vi "Graph Builder GUI - 4Dsupported.vi"() -> ()   [LabVIEW 2019]
uses:
  AxisMenu--Enum.ctl
  <vilib>/Utility/file.llb/Read Delimited Spreadsheet (string).vi
panel:
  in  "Axis Menus 2":T1={"Axis Menu 1"=1, "Axis Menu 2"=3, "Axis Menu 3"=0, "Axis Menu 4"=7, "Axis Menu 5"=9, "Axis Menu 6"=0, "Axis Menu 7"=0, "Axis Menu 8"=0, "Axis Menu 9"=4, "Axis Menu 10"=2, "Axis Menu 11"=0, "Axis Menu 12"=0} {"Axis Menu 12" items=["test", "what", "ok"]; "Axis Menu 11" items=["<Ignore>", "<X Axis>", "<Y Axis>", "<Color Axis>", "<Time Axis>", "<Supra-X Scroll>", "<Supra-Y Scroll>", "0.130833", "0.130832", "0.130830", "0.130828", "0.130824", "0.130816", "0.130803", "0.130780", "0.130738", "0.130664", "0.130532", "0.148603", "0.148602", "0.148601", "0.148600", "0.148597", "0.148593", "0.148584", "0.148569", "0.148542", "0.148495", "0.148411", "0.148262", "0.169040", "0.169039", "0.169038", "0.169036", "0.169033", "0.169028", "0.169018", "0.169001", "0.168971", "0.168917", "0.168821", "0.168651", "0.191677", "0.191676", "0.191675", "0.191674", "0.191672", "0.191669", "0.191663", "0.191652", "0.191633", "0.191598", "0.191537", "0.191429", "0.191236", "0.216833", "0.216832", "0.216831", "0.216828", "0.216824", "0.216818", "0.216805", "0.216783", "0.216745", "0.216676", "0.216553", "0.216335", "0.247333", "0.247332", "0.247330", "0.247328", "0.247323", "0.247315", "0.247301", "0.247276", "0.247232", "0.247153", "0.247013", "0.246764", "0.282147", "0.282146", "0.282145", "0.282143", "0.282140", "0.282135", "0.282126", "0.282110", "0.282082", "0.282031", "0.281941", "0.281782", "0.281498", "0.132273", "0.132272", "0.132270", "0.132268", "0.132264", "0.132256", "0.132243", "0.132219", "0.132177", "0.132102", "0.131969", "0.150477", "0.150476", "0.150475", "0.150473"]; "Axis Menu 10" items=["<Ignore>", "<X Axis>", "<Y Axis>", "<Color Axis>", "<Time Axis>", "<Supra-X Scroll>", "<Supra-Y Scroll>", " 0.000001", " 0.000100", " 0.000178", " 0.000316", " 0.000562", " 0.001000", " 0.001778", " 0.003162", " 0.005623", " 0.010000", " 0.017783", " 0.031623", " 0.056234", " 0.100000", " 0.177828", " 0.316228", " 0.562341", " 1.000000", " 1.778279", " 3.162278", " 5.623413", " 10.000000"]; "Axis Menu 9" items=["<Ignore>", "<X Axis>", "<Y Axis>", "<Color Axis>", "<Time Axis>", "<Supra-X Scroll>", "<Supra-Y Scroll>", "0.000000", "0.000009", "0.000008", "0.000007", "0.000027", "0.000026", "0.000024", "0.000023", "0.000021", "0.000020", "0.000019", "0.009968", "0.011864", "0.014201", "0.017147", "0.020963", "0.026238", "0.033996", "0.021918", "0.023911", "0.025861", "0.026573", "0.030301", "0.047063", "0.057440", "0.023065", "0.025858", "0.047064", "0.023066", "0.030300", "0.043640", "0.041839", "0.040309", "0.039572", "0.040076", "0.047266", "0.070634", "0.043275", "0.041840", "0.040209", "0.039424", "0.047267", "0.040077", "0.068931", "0.041841", "0.039425", "0.041842", "0.040188", "0.057164", "0.055857", "0.053803", "0.064045", "0.062643", "0.079336", "0.084486", "0.057166", "0.055755", "0.053805", "0.062858", "0.062644", "0.079293", "0.084489", "0.057168", "0.055757", "0.053806", "0.062859", "0.084490", "0.057169", "0.054590", "0.053808", "0.062861", "0.062645", "0.084487", "0.057171", "0.054591", "0.053809", "0.079294", "0.084488", "0.094881", "0.146114", "0.159443", "0.157470", "0.165770", "0.210973", "0.222273", "0.083860", "0.145194", "0.159522", "0.153900", "0.165858", "0.198740", "0.221867", "0.083920", "0.145042", "0.159585", "0.153985", "0.165272", "0.198828", "0.221738", "0.083830"]; "Axis Menu 8" items=["<Ignore>", "<X Axis>", "<Y Axis>", "<Color Axis>", "<Time Axis>", "<Supra-X Scroll>", "<Supra-Y Scroll>", "0.000100", "0.115754", "0.118456", "0.121668", "0.125585", "0.130445", "0.136809", "0.145589", "0.115756", "0.118488", "0.121728", "0.125684", "0.130588", "0.137092", "0.145948", "0.115755", "0.118457", "0.121725", "0.130587", "0.137090", "0.145946", "0.130586", "0.145945", "0.125683", "0.121724", "0.130585", "0.137089", "0.116301", "0.118995", "0.122196", "0.125991", "0.130788", "0.137250", "0.146371", "0.116271", "0.118994", "0.122182", "0.125976", "0.130786", "0.137248", "0.146369", "0.125975", "0.130785", "0.137246", "0.146312", "0.118993", "0.125974", "0.137245", "0.122177", "0.130784", "0.116417", "0.119132", "0.122246", "0.126270", "0.131185", "0.137848", "0.146643", "0.119115", "0.122243", "0.126211", "0.131183", "0.137836", "0.146636", "0.116416", "0.119113", "0.126209", "0.137835", "0.146632", "0.119058", "0.122241", "0.126208", "0.131182", "0.146628", "0.116415", "0.119057", "0.126207", "0.137833", "0.146627", "0.119561", "0.123571", "0.127830", "0.132135", "0.138249", "0.146742", "0.157620", "0.119287", "0.123423", "0.127757", "0.131884", "0.138171", "0.146298", "0.157507", "0.119274", "0.123353", "0.127748", "0.131866", "0.138073", "0.146278", "0.157425", "0.119234"]; "Axis Menu 7" items=["<Ignore>", "<X Axis>", "<Y Axis>", "<Color Axis>", "<Time Axis>", "<Supra-X Scroll>", "<Supra-Y Scroll>", "39250.000000", "44581.000000", "50712.000000", "57503.000000", "65050.000000", "74200.000000", "84644.000000", "39682.000000", "45143.000000", "51191.000000", "57807.000000", "65518.000000", "74460.000000", "84954.000000", "39551.000000", "45105.000000", "51201.000000", "57817.000000", "65260.000000", "74304.000000", "84692.000000", "39877.000000", "45240.000000", "51394.000000", "58153.000000", "65752.000000", "74616.000000", "85111.000000", "39561.000000", "45096.000000", "51328.000000", "57851.000000", "65269.000000", "74275.000000", "84761.000000", "39440.000000", "44789.000000", "50739.000000", "57377.000000", "64848.000000", "73617.000000", "84298.000000", "39725.000000", "45219.000000", "51293.000000", "57890.000000", "65468.000000", "74547.000000", "85034.000000", "39753.000000", "45230.000000", "51299.000000", "58146.000000", "65861.000000", "74815.000000", "85419.000000", "39615.000000", "45004.000000", "51015.000000", "57909.000000", "65576.000000", "74531.000000", "85128.000000", "39612.000000", "44999.000000", "51011.000000", "65574.000000", "74528.000000", "85125.000000", "44998.000000", "65573.000000", "74527.000000", "85124.000000", "44997.000000", "51010.000000", "57907.000000", "65572.000000", "51009.000000", "65571.000000", "74526.000000", "39556.000000", "45059.000000", "51216.000000", "57906.000000", "65525.000000", "74511.000000", "85154.000000", "45056.000000", "51213.000000", "57901.000000", "65522.000000", "74506.000000", "85151.000000", "45055.000000", "57899.000000", "65519.000000", "74502.000000", "85145.000000", "45054.000000", "57897.000000"]; "Axis Menu 6" items=["<Ignore>", "<X Axis>", "<Y Axis>", "<Color Axis>", "<Time Axis>", "<Supra-X Scroll>", "<Supra-Y Scroll>", "1.000", "1.500", "2.000", "2.500", "3.000"]; "Axis Menu 5" items=["<Ignore>", "<X Axis>", "<Y Axis>", "<Color Axis>", "<Time Axis>", "<Supra-X Scroll>", "<Supra-Y Scroll>", "0.900", "0.950", "1.000", "1.050", "1.100", "1.150", "1.200"]; "Axis Menu 4" items=["<Ignore>", "<X Axis>", "<Y Axis>", "<Color Axis>", "<Time Axis>", "<Supra-X Scroll>", "<Supra-Y Scroll>", "300000"]; "Axis Menu 3" items=["<Ignore>", "<X Axis>", "<Y Axis>", "<Color Axis>", "<Time Axis>", "<Supra-X Scroll>", "<Supra-Y Scroll>", "0.000000E+0", "1.250000E-1", "2.500000E-1", "5.000000E-1", "1.600000E+1", "4.000000E+0", "8.000000E+0", "1.000000E+0", "2.000000E+0"]; "Axis Menu 2" items=["<Ignore>", "<X Axis>", "<Y Axis>", "<Color Axis>", "<Time Axis>", "<Supra-X Scroll>", "<Supra-Y Scroll>", "1.000000E-10", "1.000000E-1", "2.000000E-1", "3.000000E-1", "4.000000E-1", "5.000000E-1", "6.000000E-1", "7.000000E-1", "8.000000E-1", "9.000000E-1", "1.000000E+0", "1.100000E+0", "1.200000E+0", "1.300000E+0", "1.400000E+0", "1.500000E+0", "1.600000E+0", "1.700000E+0", "1.800000E+0", "1.900000E+0", "2.000000E+0", "3.000000E+0", "4.000000E+0", "5.000000E+0"]; "Axis Menu 1" items=["<Ignore>", "<X Axis>", "<Y Axis>", "<Color Axis>", "<Time Axis>", "<Supra-X Scroll>", "<Supra-Y Scroll>", "SPHERE", "SLAB"]}
  out "Array":cluster{string[]}[](array[cluster])
  out "Time vs Color":T2(array[cluster])
  in  "Axis Menu Type Def":T3 caption="Axis Menu" items=["<Ignore>", "<X Axis>", "<Y Axis>", "<Color Axis>", "<Time Axis>", "<Supra-X Scroll>", "<Supra-Y Scroll>"]
  in  "Normalize? (F)":bool
  in  "Path to Cleaned Data File":path=path "D:/Dropbox/PostDoc/Programs/Data/2019-11-27 run 2020-01-02 CLEAN v06.txt"
  out "Color vs Time":T2(array[cluster])
  in  "Axis Menus 2":T1={"Axis Menu 1"=1, "Axis Menu 2"=3, "Axis Menu 3"=0, "Axis Menu 4"=7, "Axis Menu 5"=9, "Axis Menu 6"=0, "Axis Menu 7"=0, "Axis Menu 8"=0, "Axis Menu 9"=4, "Axis Menu 10"=2, "Axis Menu 11"=0, "Axis Menu 12"=0} {"Axis Menu 12" items=["test", "what", "ok"]; "Axis Menu 11" items=["<Ignore>", "<X Axis>", "<Y Axis>", "<Color Axis>", "<Time Axis>", "<Supra-X Scroll>", "<Supra-Y Scroll>", "0.124790", "0.124789", "0.124788", "0.124787", "0.149483", "0.149482", "0.149481", "0.149480", "0.170070", "0.170069", "0.170068", "0.170066", "0.181603", "0.181602", "0.181601", "0.181599", "0.218283", "0.218282", "0.218281", "0.218278", "0.245293", "0.245292", "0.245290", "0.245288", "0.274817", "0.274816", "0.274815", "0.274813", "0.274810", "0.125677", "0.125676", "0.125675", "0.125674", "0.150653", "0.150652", "0.150651", "0.150650", "0.171020", "0.171019", "0.171018", "0.171016", "0.182680", "0.182679", "0.182678", "0.182676", "0.219353", "0.219352", "0.219350", "0.219348", "0.245337", "0.245336", "0.245335", "0.245333", "0.245331", "0.275040", "0.275039", "0.275038", "0.275036", "0.275034", "0.125530", "0.125529", "0.125528", "0.125527", "0.150820", "0.150819", "0.150818", "0.150817", "0.171260", "0.171259", "0.171258", "0.171256", "0.182963", "0.182962", "0.182961", "0.182959", "0.219583", "0.219582", "0.219580", "0.219578", "0.245663", "0.245662", "0.245660", "0.245658", "0.275477", "0.275476", "0.275475", "0.275473", "0.275470", "0.125047", "0.125046", "0.125045", "0.125044", "0.149950", "0.149949", "0.149948", "0.149947", "0.170673", "0.170672", "0.170671", "0.170669"]; "Axis Menu 10" items=["<Ignore>", "<X Axis>", "<Y Axis>", "<Color Axis>", "<Time Axis>", "<Supra-X Scroll>", "<Supra-Y Scroll>", " 0.000001", " 0.000100", " 0.000178", " 0.000316", " 0.000562", " 0.001000", " 0.001778", " 0.003162", " 0.005623", " 0.010000", " 0.017783", " 0.031623", " 0.056234", " 0.100000", " 0.177828", " 0.316228", " 0.562341", " 1.000000", " 1.778279", " 3.162278", " 5.623413", " 10.000000"]; "Axis Menu 9" items=["<Ignore>", "<X Axis>", "<Y Axis>", "<Color Axis>", "<Time Axis>", "<Supra-X Scroll>", "<Supra-Y Scroll>", "0.101993", "0.096633", "0.092658", "0.085990", "0.075300", "0.059477", "0.039123", "0.018608", "0.004991", "0.000489", "0.000008", "0.000000", "0.116800", "0.110554", "0.105927", "0.098173", "0.085768", "0.067469", "0.044068", "0.020714", "0.005453", "0.000520", "0.000009", "0.132927", "0.125677", "0.120312", "0.111335", "0.097004", "0.075951", "0.049213", "0.022829", "0.005889", "0.000546", "0.151310", "0.142863", "0.136620", "0.126191", "0.109591", "0.085325", "0.054762", "0.025015", "0.006305", "0.000568", "0.171807", "0.161952", "0.154680", "0.142557", "0.123328", "0.095386", "0.060546", "0.027176", "0.006681", "0.000585", "0.194440", "0.182929", "0.174453", "0.160356", "0.138091", "0.105973", "0.066407", "0.029225", "0.006998", "0.000597", "0.220313", "0.206759", "0.196805", "0.180303", "0.154383", "0.117340", "0.072403", "0.031148", "0.007253", "0.000604", "0.249937", "0.233807", "0.222004", "0.202522", "0.172147", "0.129274", "0.078287", "0.032824", "0.007433", "0.000607", "0.284960", "0.265378", "0.251127", "0.227750", "0.191693", "0.141694", "0.083838", "0.034153", "0.007539", "0.000608", "0.099317", "0.094097", "0.090227", "0.083736", "0.073333", "0.057935", "0.038123"]; "Axis Menu 8" items=["<Ignore>", "<X Axis>", "<Y Axis>", "<Color Axis>", "<Time Axis>", "<Supra-X Scroll>", "<Supra-Y Scroll>", " 0.000000", " 0.010000", " 0.017783", " 0.031623", " 0.056234", " 0.100000", " 0.177828", " 0.316228", " 0.562341", " 1.000000", " 1.778279", " 3.162278", " 5.623413", " 10.000000"]; "Axis Menu 7" items=["<Ignore>", "<X Axis>", "<Y Axis>", "<Color Axis>", "<Time Axis>", "<Supra-X Scroll>", "<Supra-Y Scroll>", "0.151508", "0.180212", "0.214514", "0.257326", "0.309635", "0.375025", "0.461527", "0.581184", "0.760931", "0.250173", "0.276650", "0.305752", "0.353413", "0.398546", "0.442409", "0.520362", "0.657056", "0.827587", "0.414001", "0.407660", "0.414563", "0.447402", "0.466145", "0.504594", "0.582028", "0.704423", "0.867666", "0.433548", "0.634418", "0.628125", "0.628008", "0.641001", "0.657422", "0.709239", "0.825406", "0.993748", "0.373263", "0.432931", "0.449074", "0.489411", "0.516368", "0.660312", "0.724828", "0.968868", "1.088399", "0.335947", "0.367037", "0.394834", "0.443654", "0.514408", "0.554588", "0.641080", "0.735371", "0.910263", "0.327704", "0.332848", "0.414185", "0.467251", "0.480735", "0.556127", "0.623152", "0.699726", "0.859418", "0.461173", "0.491789", "0.501993", "0.590991", "0.610121", "0.723825", "0.769819", "0.890022", "1.039443", "0.882501", "0.905582", "0.883806", "0.907114", "0.895778", "0.939819", "0.999607", "1.087521", "1.200907", "0.781780", "0.881722", "0.877851", "0.868481", "0.886882", "0.925460", "0.984676", "1.102925", "1.216024", "0.566459", "0.555943", "0.726802", "0.796129", "0.880437", "0.915396", "0.953298", "1.049153", "1.205753", "0.347360"]; "Axis Menu 6" items=["<Ignore>", "<X Axis>", "<Y Axis>", "<Color Axis>", "<Time Axis>", "<Supra-X Scroll>", "<Supra-Y Scroll>", "2.344834", "2.387126", "2.436041", "2.495505", "2.566510", "2.651930", "2.760088", "2.901185", "3.098524", "2.345382", "2.387759", "2.437268", "2.493627", "2.563980", "2.648439", "2.753246", "2.894023", "3.089221", "2.352875", "2.394568", "2.444453", "2.502000", "2.572868", "2.658786", "2.765348", "2.908156", "3.107787", "2.357135", "2.401976", "2.452351", "2.509386", "2.581015", "2.667360", "2.775665", "2.921966", "3.124767", "2.355467", "2.398480", "2.448976", "2.506777", "2.578139", "2.666193", "2.774983", "2.921659", "3.124084", "2.353391", "2.396340", "2.447023", "2.504390", "2.576456", "2.662857", "2.771609", "2.915206", "3.116901", "2.347116", "2.388769", "2.439723", "2.498575", "2.566889", "2.651012", "2.756869", "2.895103", "3.086171", "2.358209", "2.402290", "2.452409", "2.511872", "2.583080", "2.670274", "2.778499", "2.921880", "3.121392", "2.376488", "2.420674", "2.469871", "2.529509", "2.599974", "2.687483", "2.798687", "2.944386", "3.148969", "2.371796", "2.417104", "2.468122", "2.527208", "2.598433", "2.685195", "2.795190", "2.942178", "3.147741", "2.366926", "2.408807", "2.461273", "2.522342", "2.595422", "2.681896", "2.790502", "2.936582", "3.141625", "2.348115"]; "Axis Menu 5" items=["<Ignore>", "<X Axis>", "<Y Axis>", "<Color Axis>", "<Time Axis>", "<Supra-X Scroll>", "<Supra-Y Scroll>", "30598.000000", "35040.000000", "39878.000000", "45393.000000", "51542.000000", "58332.000000", "66094.000000", "74981.000000", "85488.000000", "29795.000000", "34184.000000", "39037.000000", "44238.000000", "50281.000000", "57032.000000", "64585.000000", "73380.000000", "83883.000000", "30215.000000", "34598.000000", "39529.000000", "44781.000000", "50906.000000", "57711.000000", "65300.000000", "74207.000000", "84839.000000", "30420.000000", "34848.000000", "39820.000000", "45093.000000", "51234.000000", "58058.000000", "65731.000000", "74738.000000", "85412.000000", "30346.000000", "34780.000000", "39755.000000", "44993.000000", "51134.000000", "57949.000000", "65619.000000", "74607.000000", "85278.000000", "30271.000000", "34685.000000", "39667.000000", "44889.000000", "50998.000000", "57803.000000", "65475.000000", "74451.000000", "85086.000000", "28988.000000", "33307.000000", "38089.000000", "43442.000000", "49401.000000", "55907.000000", "63461.000000", "72313.000000", "82618.000000", "29702.000000", "34099.000000", "38944.000000", "44333.000000", "50383.000000", "56996.000000", "64669.000000", "73617.000000", "84134.000000", "30102.000000", "34552.000000", "39426.000000", "44865.000000", "50933.000000", "57617.000000", "65344.000000", "74404.000000", "85097.000000", "29976.000000", "34421.000000", "39306.000000", "44726.000000", "50780.000000", "57419.000000", "65105.000000", "74181.000000", "84902.000000", "29837.000000", "34242.000000", "39137.000000", "44539.000000", "50553.000000", "57221.000000", "64866.000000", "73902.000000", "84610.000000", "28547.000000"]; "Axis Menu 4" items=["<Ignore>", "<X Axis>", "<Y Axis>", "<Color Axis>", "<Time Axis>", "<Supra-X Scroll>", "<Supra-Y Scroll>", "1.000", "1.500", "2.000", "2.500", "3.000"]; "Axis Menu 3" items=["<Ignore>", "<X Axis>", "<Y Axis>", "<Color Axis>", "<Time Axis>", "<Supra-X Scroll>", "<Supra-Y Scroll>", "0.800", "0.850", "0.900", "0.950", "1.000", "1.050", "1.100", "1.150", "1.200"]; "Axis Menu 2" items=["<Ignore>", "<X Axis>", "<Y Axis>", "<Color Axis>", "<Time Axis>", "<Supra-X Scroll>", "<Supra-Y Scroll>", "0.000000E+0", "1.000000E-1", "1.778279E-1", "3.162278E-1", "5.623413E-1", "1.000000E+0", "1.778279E+0", "1.000000E+1", "3.162278E+0", "5.623413E+0"]; "Axis Menu 1" items=["<Ignore>", "<X Axis>", "<Y Axis>", "<Color Axis>", "<Time Axis>", "<Supra-X Scroll>", "<Supra-Y Scroll>", "2.100000E+0", "2.200000E+0", "2.300000E+0", "2.400000E+0", "2.600000E+0", "2.700000E+0", "2.800000E+0", "2.900000E+0", "1.000000E-9", "1.000000E-1", "2.000000E-1", "3.000000E-1", "4.000000E-1", "5.000000E-1", "6.000000E-1", "7.000000E-1", "8.000000E-1", "9.000000E-1", "1.000000E+0", "1.100000E+0", "1.200000E+0", "1.300000E+0", "1.400000E+0", "1.500000E+0", "1.600000E+0", "1.700000E+0", "1.800000E+0", "1.900000E+0", "2.000000E+0", "2.500000E+0", "3.000000E+0", "3.500000E+0", "4.000000E+0", "4.500000E+0", "5.000000E+0"]}
  in  "Color 1":u32(colorbox)
  in  "Color 2":u32(colorbox)=16711680
  # "D:\\Dropbox\\PostDoc\\Programs\\Data\\2018-09-18 2020-01-03 newResults v02 -- CLEAN3.txt"
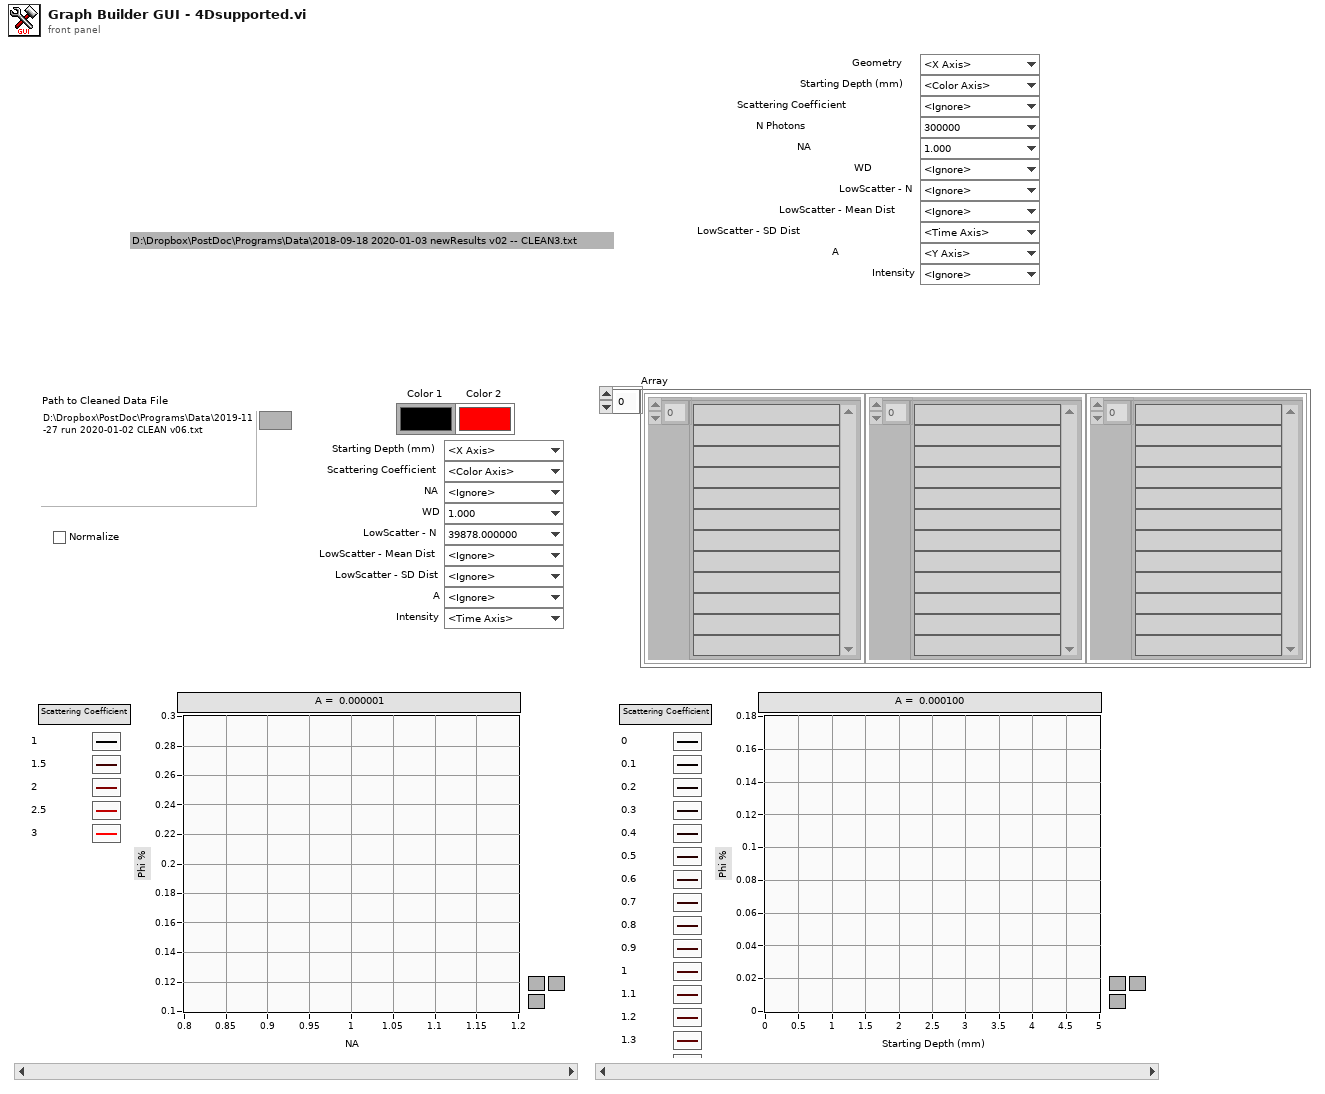
[diagram p1: front panel]
types:
  T1 = cluster{"Axis Menu 1":u16, "Axis Menu 2":u16, "Axis Menu 3":u16, "Axis Menu 4":u16, "Axis Menu 5":u16, "Axis Menu 6":u16, "Axis Menu 7":u16, "Axis Menu 8":u16, "Axis Menu 9":u16, "Axis Menu 10":u16, "Axis Menu 11":u16, "Axis Menu 12":u16}
  T2 = cluster{"XY Graph in Array":cluster{dbl[], dbl[]}[], "String":string, "String 2":string}[]
  T3 = typedef "AxisMenu--Enum.ctl" = u16
  T4 = cluster{cluster{dbl[], dbl[]}[], string, "Caption.Text":string}[]
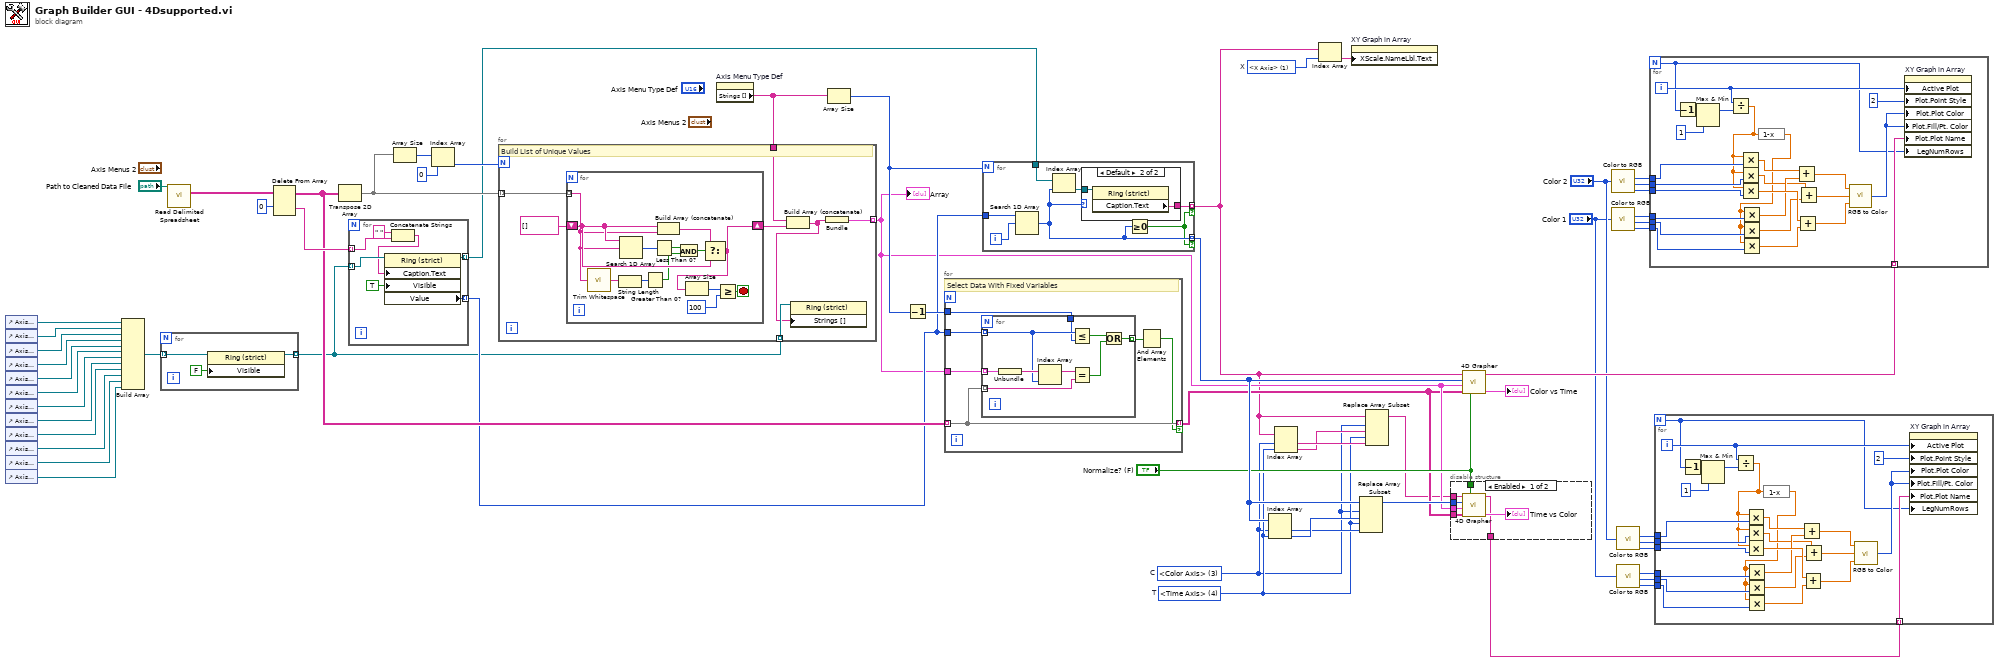
[diagram p0: block diagram]
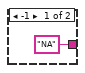
[diagram p3: hidden frame]
diagram:
  w13 = T3 4 items=["<Ignore>", "<X Axis>", "<Y Axis>", "<Color Axis>", "<Time Axis>", "<Supra-X Scroll>", "<Supra-Y Scroll>"]  # T
  w12 = T3 3 items=["<Ignore>", "<X Axis>", "<Y Axis>", "<Color Axis>", "<Time Axis>", "<Supra-X Scroll>", "<Supra-Y Scroll>"]  # C
  w27 = T3 1 items=["<Ignore>", "<X Axis>", "<Y Axis>", "<Color Axis>", "<Time Axis>", "<Supra-X Scroll>", "<Supra-Y Scroll>"]  # X
  n1 = control-ref of="Axis Menu 1"() -> (w33:refnum<vi>)
  n2 = control-ref of="Axis Menu 2"() -> (w49:refnum<vi>)
  n3 = control-ref of="Axis Menu 3"() -> (w48:refnum<vi>)
  n4 = control-ref of="Axis Menu 4"() -> (w47:refnum<vi>)
  n5 = control-ref of="Axis Menu 5"() -> (w46:refnum<vi>)
  n6 = control-ref of="Axis Menu 6"() -> (w45:refnum<vi>)
  n7 = control-ref of="Axis Menu 7"() -> (w44:refnum<vi>)
  n8 = control-ref of="Axis Menu 8"() -> (w43:refnum<vi>)
  n9 = control-ref of="Axis Menu 9"() -> (w42:refnum<vi>)
  n10 = control-ref of="Axis Menu 10"() -> (w41:refnum<vi>)
  n11 = control-ref of="Axis Menu 11"() -> (w40:refnum<vi>)
  n12 = control-ref of="Axis Menu 12"() -> (w39:refnum<vi>)
  n13 = Build Array(w33, w49, w48, w47, w46, w45, w44, w43, w42, w41, w40, w39) -> (w37:refnum<vi>[])
  n14 = for {
    tunnel: w37 -> [w63] mode=indexing
    tunnel: [w61] -> w25 mode=indexing
    n15 = property on="Property Node" class="Ring (strict)"(reference=w63, "Visible"=FALSE) -> (reference out=w61:refnum<vi>)  [unwired: 1 in, 1 out]
  }
  n16 = call-poly <vilib>:"Read Delimited Spreadsheet.vi"("file path (dialog if empty)"="Path to Cleaned Data File") -> ("all rows"=w34:string[][])  [unwired: 9 in, 5 out]
  n17 = Delete From Array(array=w34, index (row)=0) -> (deleted portion=w38:string[], array with subset deleted=w32:string[][])  [unwired: 2 in]
  n18 = Transpose 2D Array(2D array=w32) -> (transposed array=w58:string[][])
  n19 = for {
    tunnel: w38 -> [w66] mode=indexing
    tunnel: w25 -> [w70] mode=indexing
    tunnel: [w68] -> w29 mode=indexing
    tunnel: [w67] -> w26 mode=indexing
    n20 = Concatenate Strings(" " ("string"), w66) -> (w64:string)
    n21 = property on="Property Node" class="Ring (strict)"(reference=w70, "Caption.Text"=w64, "Visible"=TRUE) -> (reference out=w67:refnum<vi>, "Value"=w68:u16)  [unwired: 1 in, 1 out]
  }
  n22 = Array Size(array=w58) -> (size(s)=w59:i32[])
  n23 = Index Array(array=w59, index=0) -> (element=w36:i32)
  n24 = property on="Axis Menu Type Def" class="Ring (strict)"() -> ("Strings []"=w31:string[])  [unwired: 2 in, 2 out]
  n25 = for {
    N: w36 -> [_]
    tunnel: w58 -> [w77] mode=indexing
    tunnel: [w75] -> w17 mode=indexing
    tunnel: w31 -> [w74]
    tunnel: w25 -> [w73] mode=indexing
    # "Build List of Unique Values"
    n26 = for {
      tunnel: w77 -> [w79] mode=indexing
      shift-right: [w86] -> w71
      shift-left: string[] [] -> [w90]
      stop <- w83 stop-if-true
      n27 = call <vilib>:"Trim Whitespace.vi"("string"=w79) -> ("trimmed string"=w78:string)  [unwired: 1 in]
      n28 = String Length(string=w78) -> (length=w82:i32)
      n29 = Search 1D Array(1D array=w90, element=w79) -> (index of element=w88:i32)  [unwired: 1 in]
      n30 = Greater Than 0?(x=w82) -> (x > 0?=w80:bool)
      n31 = Less Than 0?(x=w88) -> (x < 0?=w87:bool)
      n32 = Build Array (concatenate)(w90, w79) -> (w89:string[])
      n33 = And(x=w87, y=w80) -> (x .and. y?=w81:bool)
      n34 = Select(t=w89, s=w81, f=w90) -> (s? t:f=w86:string[])
      n35 = Array Size(array=w86) -> (size(s)=w85:i32)
      n36 = Greater Or Equal?(x=w85, y=100) -> (x >= y?=w83:bool)
    }
    n37 = Build Array (concatenate)(w74, w71) -> (w72:string[])
    n38 = property on="Property Node" class="Ring (strict)"(reference=w73, "Strings []"=w72) -> ()  [unwired: 1 in, 2 out]
    n39 = Bundle(w72) -> (w75:cluster{string[]})  [unwired: 1 in]
  }
  "Array" <- w17
  n40 = Array Size(array=w31) -> (size(s)=w24:i32)
  n41 = Decrement(x=w24) -> (x-1=w30:i32)
  n42 = for {
    tunnel: w32 -> [w95] mode=indexing
    tunnel: [w95] -> w16 mode=indexing if=w92
    tunnel: w29 -> [w96]
    tunnel: w17 -> [w94]
    tunnel: w30 -> [w91]
    # "Select Data With Fixed Variables"
    n43 = for {
      tunnel: w96 -> [w101] mode=indexing
      tunnel: w95 -> [w103] mode=indexing
      tunnel: w94 -> [w105] mode=indexing
      tunnel: [w98] -> w93 mode=indexing
      tunnel: w91 -> [w97]
      n44 = Unbundle(w105) -> (w104:string[])
      n45 = Index Array(array=w104, index=w101) -> (element=w102:string)
      n46 = Less Or Equal?(x=w101, y=w97) -> (x <= y?=w100:bool)
      n47 = Equal?(x=w102, y=w103) -> (x = y?=w99:bool)
      n48 = Or(x=w100, y=w99) -> (x .or. y?=w98:bool)
    }
    n49 = And Array Elements(Boolean array=w93) -> (logical AND=w92:bool)
  }
  n50 = for {
    N: w24 -> [_]
    tunnel: w29 -> [w112]
    tunnel: [w107] -> w22 mode=indexing if=w106
    tunnel: w26 -> [w109]
    tunnel: [w108] -> w11 mode=indexing if=w106
    i -> [w111]
    n51 = Search 1D Array(1D array=w112, element=w111) -> (index of element=w107:i32)  [unwired: 1 in]
    n52 = Index Array(array=w109, index=w107) -> (element=w110:refnum<vi>)
    n53 = case shown="Default" w107 {
      tunnel: w110 -> [_ w115]
      tunnel: ["NA" ("Caption.Text") w114] -> w108
      frame -1 {
      }
      frame Default {
        n54 = property on="Property Node" class="Ring (strict)"(reference=w115) -> ("Caption.Text"=w114:string)  [unwired: 1 in, 2 out]
      }
    }
    n55 = Greater Or Equal To 0?(x=w107) -> (x >= 0?=w106:bool)
  }
  n56 = Index Array(array=w22, index #1=w12, index #2=w13) -> (element #1=w20:i32, element #2=w21:i32)
  n57 = Index Array(array=w11, index #1=w12, index #2=w13) -> (element #1=w15:string, element #2=w14:string)
  n58 = Index Array(array=w11, index=w27) -> (element=w28:string)
  n59 = property on="XY Graph in Array" class="XYGraph (strict)"("XScale.NameLbl.Text"=w28) -> ()  [unwired: 2 in, 2 out]
  n60 = Replace Array Subset(array=w22, new element #1=w21, index #1=w12, new element #2=w20, index #2=w13) -> (w19:i32[])
  n61 = Replace Array Subset(array=w11, new element #1=w14, index #1=w12, new element #2=w15, index #2=w13) -> (w10:string[])
  n62 = disable-structure shown="Enabled" {
    disable-tunnel: w19 -> [w122 _]
    disable-tunnel: "Normalize? (F)" -> [w121 _]
    disable-tunnel: w17 -> [w120 _]
    disable-tunnel: w16 -> [w119 _]
    disable-tunnel: w10 -> [w117 _]
    disable-tunnel: [w116 _] -> w3
    frame Enabled {
      n63 = call "4D Grapher.vi"("Normalize? (F)"=w121, "Pruned Data"=w119, "String Items from Axes Menus"=w120, "Axes Indexes"=w122, "Axes Names"=w117) -> ("Graph"=→"Time vs Color":T4, "Color Axis Titles"=w116:string[])  [unwired: 5 in]
    }
    frame Disabled {
    }
  }
  n64 = call "4D Grapher.vi"("Normalize? (F)"="Normalize? (F)", "Pruned Data"=w16, "String Items from Axes Menus"=w17, "Axes Indexes"=w22, "Axes Names"=w11) -> ("Graph"=→"Color vs Time":T4, "Color Axis Titles"=w50:string[])  [unwired: 5 in]
  n65 = call <vilib>:"Color to RGB.vi"("Color"="Color 2") -> ("R"=w56:u8, "G"=w55:u8, "B"=w54:u8)  [unwired: 1 out]
  n66 = call <vilib>:"Color to RGB.vi"("Color"="Color 1") -> ("R"=w53:u8, "G"=w52:u8, "B"=w51:u8)  [unwired: 1 out]
  n67 = call <vilib>:"Color to RGB.vi"("Color"="Color 2") -> ("R"=w4:u8, "G"=w5:u8, "B"=w6:u8)  [unwired: 1 out]
  n68 = call <vilib>:"Color to RGB.vi"("Color"="Color 1") -> ("R"=w7:u8, "G"=w8:u8, "B"=w9:u8)  [unwired: 1 out]
  n69 = for {
    N -> [w125]
    tunnel: w56 -> [w144]
    tunnel: w55 -> [w143]
    tunnel: w54 -> [w142]
    tunnel: w53 -> [w141]
    tunnel: w52 -> [w140]
    tunnel: w51 -> [w139]
    tunnel: w50 -> [w126] mode=indexing
    i -> [w146]
    n70 = Decrement(x=w125) -> (x-1=w145:i32)
    n71 = Max & Min(x=w145, y=1) -> (max(x,y)=w124:i32)  [unwired: 1 out]
    n72 = Divide(x=w146, y=w124) -> (x/y=w138:dbl)
    n73 = Multiply(x=w138, y=w144) -> (x*y=w132:dbl)
    n74 = Multiply(x=w138, y=w143) -> (x*y=w133:dbl)
    n75 = Multiply(x=w138, y=w142) -> (x*y=w136:dbl)
    n76 = expression code="1-x"(w138) -> (w128:dbl)
    n77 = Multiply(x=w128, y=w141) -> (x*y=w134:dbl)
    n78 = Multiply(x=w128, y=w140) -> (x*y=w135:dbl)
    n79 = Multiply(x=w128, y=w139) -> (x*y=w137:dbl)
    n80 = Add(x=w132, y=w134) -> (x+y=w131:dbl)
    n81 = Add(x=w136, y=w137) -> (x+y=w129:dbl)
    n82 = Add(x=w133, y=w135) -> (x+y=w130:dbl)
    n83 = call <vilib>:"RGB to Color.vi"("B"=w129, "G"=w130, "R"=w131) -> ("Color"=w127:u32)
    n84 = property on="XY Graph in Array" class="XYGraph (strict)"("Active Plot"=w146, "Plot.Point Style"=u8 2, "Plot.Plot Color"=w127, "Plot.Fill/Pt. Color"=w127, "Plot.Plot Name"=w126, "LegNumRows"=w125) -> ()  [unwired: 2 in, 2 out]
  }
  n85 = for {
    N -> [w150]
    tunnel: w4 -> [w169]
    tunnel: w5 -> [w168]
    tunnel: w6 -> [w167]
    tunnel: w7 -> [w166]
    tunnel: w8 -> [w165]
    tunnel: w9 -> [w164]
    tunnel: w3 -> [w151] mode=indexing
    i -> [w171]
    n86 = Decrement(x=w150) -> (x-1=w170:i32)
    n87 = Max & Min(x=w170, y=1) -> (max(x,y)=w149:i32)  [unwired: 1 out]
    n88 = Divide(x=w171, y=w149) -> (x/y=w163:dbl)
    n89 = Multiply(x=w163, y=w169) -> (x*y=w157:dbl)
    n90 = Multiply(x=w163, y=w168) -> (x*y=w158:dbl)
    n91 = Multiply(x=w163, y=w167) -> (x*y=w161:dbl)
    n92 = expression code="1-x"(w163) -> (w153:dbl)
    n93 = Multiply(x=w153, y=w166) -> (x*y=w159:dbl)
    n94 = Multiply(x=w153, y=w165) -> (x*y=w160:dbl)
    n95 = Multiply(x=w153, y=w164) -> (x*y=w162:dbl)
    n96 = Add(x=w157, y=w159) -> (x+y=w156:dbl)
    n97 = Add(x=w161, y=w162) -> (x+y=w154:dbl)
    n98 = Add(x=w158, y=w160) -> (x+y=w155:dbl)
    n99 = call <vilib>:"RGB to Color.vi"("B"=w154, "G"=w155, "R"=w156) -> ("Color"=w152:u32)
    n100 = property on="XY Graph in Array" class="XYGraph (strict)"("Active Plot"=w171, "Plot.Point Style"=u8 2, "Plot.Plot Color"=w152, "Plot.Fill/Pt. Color"=w152, "Plot.Plot Name"=w151, "LegNumRows"=w150) -> ()  [unwired: 2 in, 2 out]
  }
